vi "arrays.vi"() -> ()   [LabVIEW 2013]
panel:
  out "Schedule 4":i32[](array[numeric])
  out "Schedule 3":i32[](array[numeric])
  out "Schedule 2":i32[](array[numeric])
  out "Schedule":i32[](array[numeric])
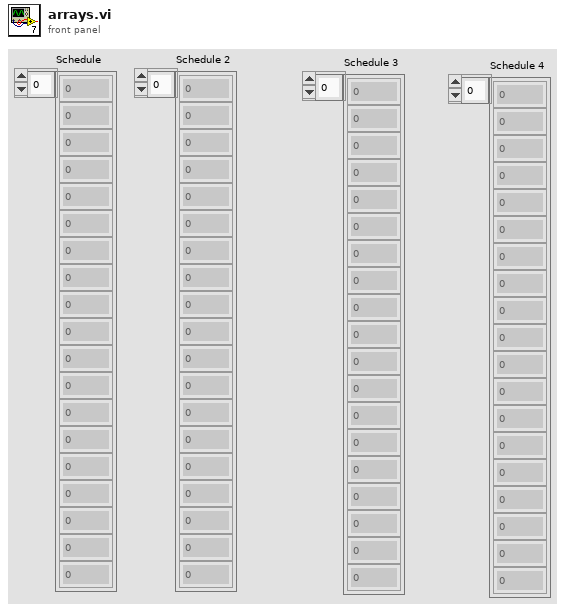
[diagram p1: front panel]
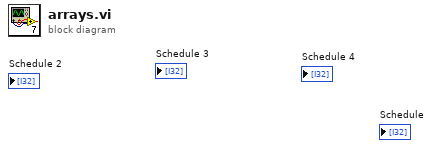
[diagram p0: block diagram]
diagram:
